vi "Query axis step amplitudes.vi"() -> ()   [LabVIEW 2016, in "Drivers.lvlib" / "Agilis.lvlib"]
uses:
  Agilis.lvlib
  Direction.ctl
panel:
  out "Amplitudes":cluster{"Neg":i32, "Pos":i32}[](array[cluster])
  in  "Port":refnum<visa-resource-name>
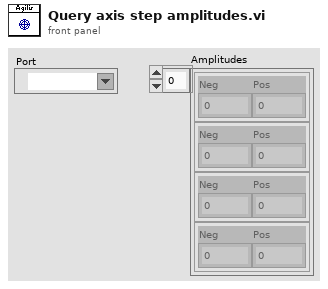
[diagram p1: front panel]
types:
  T1 = typedef "AgilisCmdLib Refnum.ctl" = refnum<k24>
  T2 = typedef "Drivers.lvlib/Agilis.lvlib/Direction.ctl" = u8
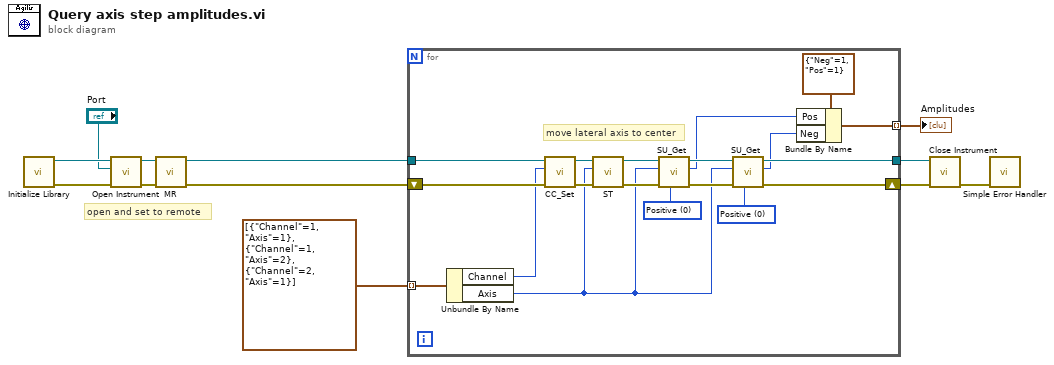
[diagram p0: block diagram]
diagram:
  # "open and set to remote"
  n1 = call "Initialize Library.vi"() -> ("error out"=w11:errorcluster, "Agilis out"=w12:T1)  [unwired: 10 in]
  n2 = call "Open Instrument.vi"("error in (no error)"=w11, "Device Key"="Port", "Agilis in"=w12) -> ("error out"=w9:errorcluster, "Agilis out"=w10:T1)  [unwired: 7 in]
  n3 = call "MR.vi"("error in (no error)"=w9, "Agilis in"=w10) -> ("error out"=w7:errorcluster, "Agilis out"=w8:T1)  [unwired: 8 in]
  n4 = for {
    tunnel: cluster{"Channel":i32, "Axis":i32}[] [{"Channel"=1, "Axis"=1}, {"Channel"=1, "Axis"=2}, {"Channel"=2, "Axis"=1}] -> [w31] mode=indexing
    tunnel: w8 -> [w30]
    shift-right: [w19] -> w3
    shift-left: w7 -> [w29]
    tunnel: [w18] -> w4
    tunnel: [w13] -> w1 mode=indexing
    w20 = T2 0 items=["Positive", "Negative"] ("Direction")
    w27 = T2 0 items=["Positive", "Negative"] ("Direction")
    # "move lateral axis to center"
    n5 = Unbundle By Name(w31) -> ("Channel"=w28:i32, "Axis"=w17:i32)
    n6 = call "CC_Set.vi"("error in (no error)"=w29, "Channel Number"=w28, "Agilis in"=w30) -> ("error out"=w25:errorcluster, "Agilis out"=w26:T1)  [unwired: 7 in]
    n7 = call "ST.vi"("error in (no error)"=w25, "Axis Number"=w17, "Agilis in"=w26) -> ("error out"=w23:errorcluster, "Agilis out"=w24:T1)  [unwired: 7 in]
    n8 = call "SU_Get.vi"("Direction"=w27, "error in (no error)"=w23, "Axis Number"=w17, "Agilis in"=w24) -> ("error out"=w21:errorcluster, "Step Amplitude"=w15:i32, "Agilis out"=w22:T1)  [unwired: 5 in]
    n9 = call "SU_Get.vi"("Direction"=w20, "error in (no error)"=w21, "Axis Number"=w17, "Agilis in"=w22) -> ("error out"=w19:errorcluster, "Step Amplitude"=w14:i32, "Agilis out"=w18:T1)  [unwired: 5 in]
    n10 = Bundle By Name(cluster=cluster{"Neg":i32, "Pos":i32} {"Neg"=1, "Pos"=1}, "Pos"=w15, "Neg"=w14) -> (w13:cluster{"Neg":i32, "Pos":i32})
  }
  "Amplitudes" <- w1
  n11 = call "Close Instrument.vi"("error in (no error)"=w3, "Agilis in"=w4) -> ("error out"=w2:errorcluster)  [unwired: 9 in]
  n12 = call <vilib>:"Simple Error Handler.vi"("error in (no error)"=w2) -> ()  [unwired: 4 in, 5 out]
